vi "square_brackets_beside_vertical_bar.vi"(8 "error in (no error)":errorcluster, 11 "Instrument Command In":string="TRIGger:AND:ENABle {{ON | 1} | {OFF | 0}} ") -> (0 "error out":errorcluster, 2 "Boolean":bool, 3 "Instrument Command Out":string)   [LabVIEW 2018]
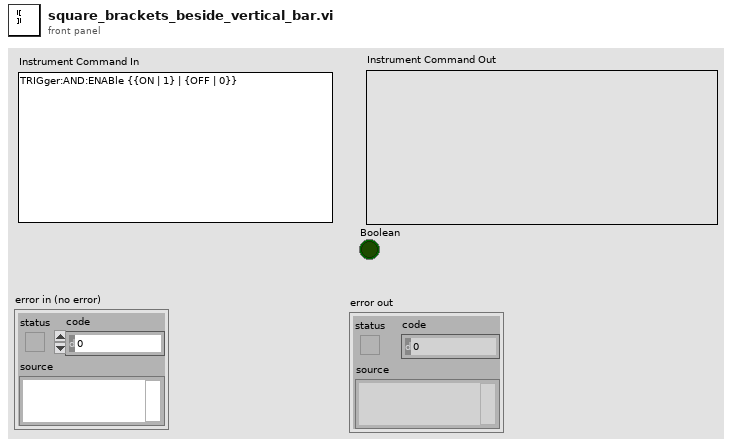
[diagram p1: front panel]
types:
  T1 = cluster{"Start Sting":string, "End String":string}
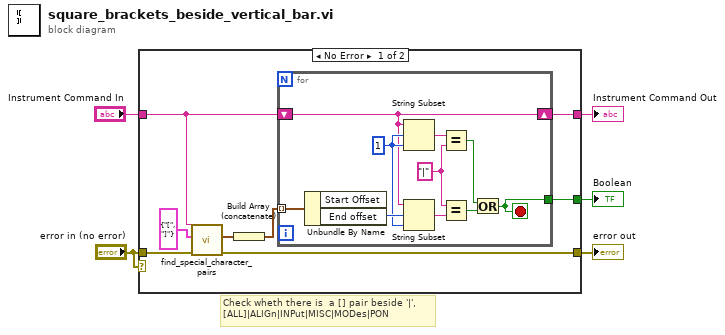
[diagram p0: block diagram]
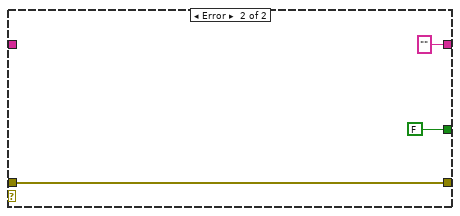
[diagram p2: hidden frame]
diagram:
  # "Check wheth there is  a [] pair beside '|', \n[ALL]|ALIGn|INPut|MISC|MODes|PON"
  n1 = case shown="No Error" "error in (no error)" {
    tunnel: [w6 "" ("result string")] -> w5
    tunnel: "Instrument Command In" -> [w8 _]
    tunnel: "error in (no error)" -> [w10 w25]
    tunnel: [w7 w25] -> w2
    tunnel: [w9 FALSE] -> w1
    frame No Error {
      n2 = call "find_special_character_pairs.vi"("error in (no error)"=w10, "String Pair"=T1 {"Start Sting"="[", "End String"="]"}, "Command String"=w8) -> ("error out"=w7:errorcluster, "Pair Offset"=w12:cluster{"Start Offset":i32, "End offset":i32}[])  [unwired: 7 out]
      n3 = Build Array (concatenate)(w12) -> (w13:cluster{"Start Offset":i32, "End offset":i32}[])
      n4 = for {
        shift-right: [w14] -> w6
        shift-left: w8 -> [w14]
        tunnel: w13 -> [w16] mode=indexing
        tunnel: [w15] -> w9
        stop <- w15 stop-if-true
        w21 = "|"
        w17 = 1
        n5 = Unbundle By Name(w16) -> ("End offset"=w18:i32)  [unwired: 1 out]
        n6 = String Subset(string=w14, offset (0)=w17, length (rest)=w17) -> (substring=w23:string)
        n7 = String Subset(string=w14, offset (0)=w18, length (rest)=w17) -> (substring=w22:string)
        n8 = Equal?(x=w23, y=w21) -> (x = y?=w20:bool)
        n9 = Equal?(x=w21, y=w22) -> (x = y?=w19:bool)
        n10 = Or(x=w20, y=w19) -> (x .or. y?=w15:bool)
      }
    }
    frame Error {
    }
  }
  "Instrument Command Out" <- w5
  "error out" <- w2
  "Boolean" <- w1
